vi "Global_linker_path_3.vi"() -> ()   [LabVIEW 2017]
panel:
  in  "LK_DB_tar":path=path "C:/BD_Monitor/LK__tareas_prog5.udl"
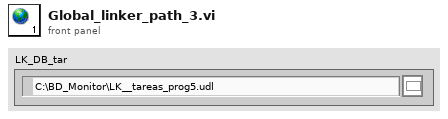
[diagram p1: front panel]
diagram:
